vi "Host Gen Trajectory.vi"(7 "Trajectory Pattern":T3(ring)=enum."Centered", 8 "Depth Ctrl Array\n(% Thickness)":dbl[](array[numeric])=[20.0, 30.0, 40.0] min=10.0 max=90.0 step=5.0 format="%#_g%%", 9 "Traj Scale Radius from Pupil Radius (Between 0 and 1)":dbl, 10 "Traj Offset from Pupil Center [mm]":dbl[](array[numeric]), 11 "SCAN_NO":string="0000") -> (0 "zVisTraj":dbl[](array[numeric]) format="%_6g", 1 "yVisTraj":dbl[](array[numeric]) format="%_6g", 2 "xVisTraj":dbl[](array[numeric]) format="%_6g")   [LabVIEW 2016]
uses:
  <vilib>/silver_ctls/ArrayMatrixCluster/Real Matrix NI_Silver.ctl
  <vilib>/Analysis/Matrix/Datatypes/RealMatrix.ctl
  <vilib>/Analysis/7linalg.llb/Real Cholesky Factorization.vi
  <vilib>/Analysis/1siggen.llb/Ramp Pattern by Samples.vi
  <vilib>/Analysis/baseanly.llb/Mean (DBL).vi
  <vilib>/Analysis/baseanly.llb/Full Cholesky Factorization.vi
  <vilib>/Analysis/baseanly.llb/Full Real Matrix Cholesky Factorization.vi
  <vilib>/Analysis/BLAS.llb/dasum - Absolute Values Sum (DBL).vi
  <vilib>/Analysis/Matrix/Numeric/Conversions/Array To Matrix - RA2.vi
  <vilib>/Analysis/NI_AALBase.lvlib
  <vilib>/gmath/NI_Gmath.lvlib
  <vilib>/Analysis/NI_AALPro.lvlib
  <vilib>/Analysis/NI_AALBLAS.lvlib
  <vilib>/Analysis/Matrix/NI_Matrix.lvlib
panel:
  out "size(s)":i32
  out "L4_out":dbl[][](array[numeric])
  out "L3_out":dbl[][](array[numeric])
  out "L2_out":dbl[][](array[numeric])
  out "L1_out":dbl[][](array[numeric])
  out "Zi":dbl[][](array[numeric])
  out "Zp":dbl[][](array[numeric])
  out "Za":dbl[][](array[numeric])
  out "Y":dbl[][](array[numeric])
  out "X":dbl[][](array[numeric])
  out "x_out":dbl[][](array[numeric])
  out "y_out":dbl[][](array[numeric])
  out "z_out":dbl[][](array[numeric])
  out "Tool Rotation":dbl[][](array[numeric])
  out "vacf_out":dbl[][](array[numeric])
  out "time (at via pts)":dbl[][](array[numeric])
  in  "Tab Control":T1(tab)
  out "zi":dbl=5.0 format="%#_3g"
  out "zp_true":dbl=5.0 format="%#_3g"
  out "zp_work":dbl=5.0 format="%#_3g"
  out "za_work":dbl=5.0 format="%#_3g"
  out "za_true":dbl=5.0 format="%#_3g"
  in  "Reflective Index":dbl=1.35 format="%#_13g"
  out "Semi-Axes [mm]":T2
  out "Lens Thickness [mm]":dbl format="%#_3g"
  out "Iris Center [mm]":dbl[](array[numeric]) format="%#_3g"
  in  "Half Span Angle":dbl=60.0
  in  "Radial Attenuation":dbl=0.2 min=0.0 max=1.0 step=0.1
  in  "XY Safety Gap [mm]":dbl=1.5 format="%#_13g"
  out "Avg Iris z_coord [mm]":dbl=-2.0 format="%#_3g"
  in  "Cycle Time [sec]":dbl[](array[numeric])=[60.0, 90.0, 120.0]
  in  "Sampling Rate [Hz]":i32=1000
  out "Za Safety Gap [mm]":dbl[](array[numeric]) format="%#_3g"
  out "Zp Safety Gap [mm]":dbl[](array[numeric]) format="%#_3g"
  in  "No. of Lobes":dbl=10.0
  in  "Radial Offset":dbl=0.2 min=0.0 max=1.0
  in  "Dist Iris2Front [mm]":dbl[](array[numeric])=[0.1, 0.1, 0.1]
  out "No. of Cycles":i32
  out "Total Time [sec]":dbl
  out "Theta1 Waveform Graph":dbl[](graph)
  out "Theta2 Waveform Graph":dbl[](graph)
  out "Theta3 Waveform Graph":dbl[](graph)
  out "Theta4 Waveform Graph":dbl[](graph)
  in  "vac_bnd":dbl[](array[numeric])=[80.0, 100.0]
  in  "z_thld":dbl[](array[numeric])=[0.5, 2.0]
  out "Vacuum Waveform Graph":dbl[](graph)
  out "Ygrid":dbl[](array[numeric])
  out "Xgrid":dbl[](array[numeric])
  in  "OCT z_orgin [mm]":dbl format="%#_13g"
  in  "OCT z_cornea [mm]":dbl format="%#_13g"
  in  "OCT z_post [mm]":dbl format="%#_13g"
  out "Trajectory Length [mm]":dbl[](array[numeric])
  out "Traj Px Waveform Graph":dbl[](graph)
  out "Traj Py Waveform Graph":dbl[](graph)
  out "Traj Pz Waveform Graph":dbl[](graph)
  out "Theta4 Overlaid":dbl[][](graph)
  out "Theta3 Overlaid":dbl[][](graph)
  out "Theta2 Overlaid":dbl[][](graph)
  out "Theta1 Overlaid":dbl[][](graph)
  # "Modify Trajectory Center and Radius"
  # "Workspace Parameters"
  # "Top View:"
  # "Cross-Sectioned View:"
  # "No-fly Zone"
  # "Entry Site Pattern"
  # "Centered Pattern"
  # "Z Workspace"
  # "Temporal"
  # "OCT Settings"
  # "XY 2D Grid"
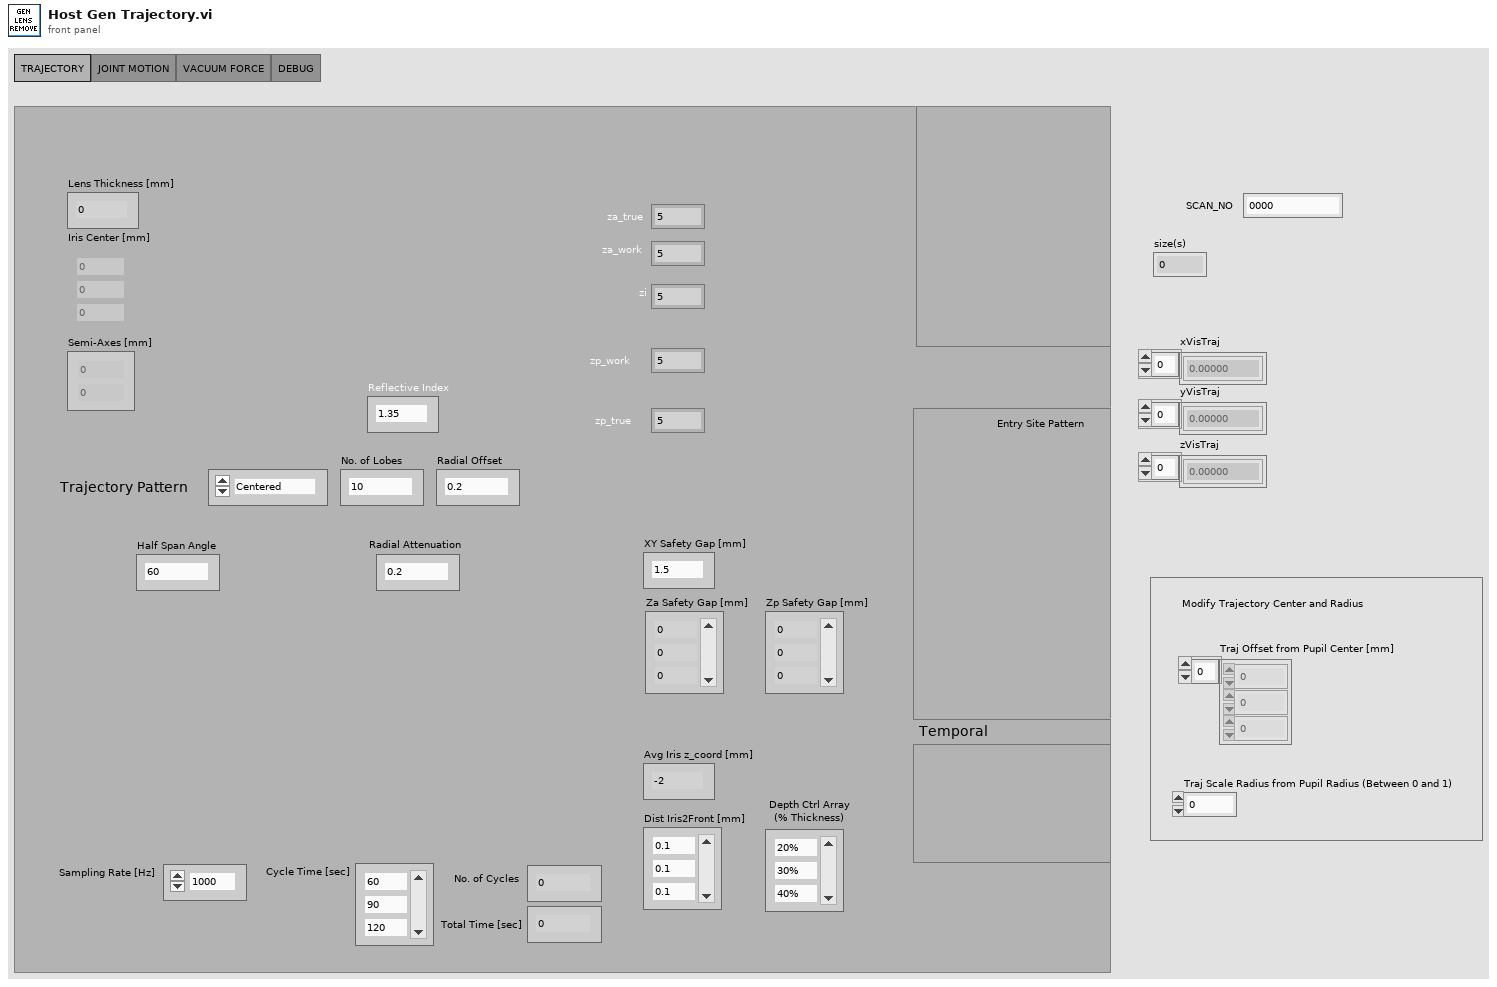
[diagram p1: front panel]
types:
  T1 = enum32{"TRAJECTORY", "JOINT MOTION", "VACUUM FORCE", "DEBUG"}
  T2 = typedef "Real Matrix NI_Silver.ctl" = dbl[][]
  T3 = enum16{"Entry Site", "Centered", "Insertion", "Extraction", "Reverse Entry Site", "Reverse Centered"}
  T4 = typedef "NI_Matrix.lvlib/RealMatrix.ctl" = dbl[][]
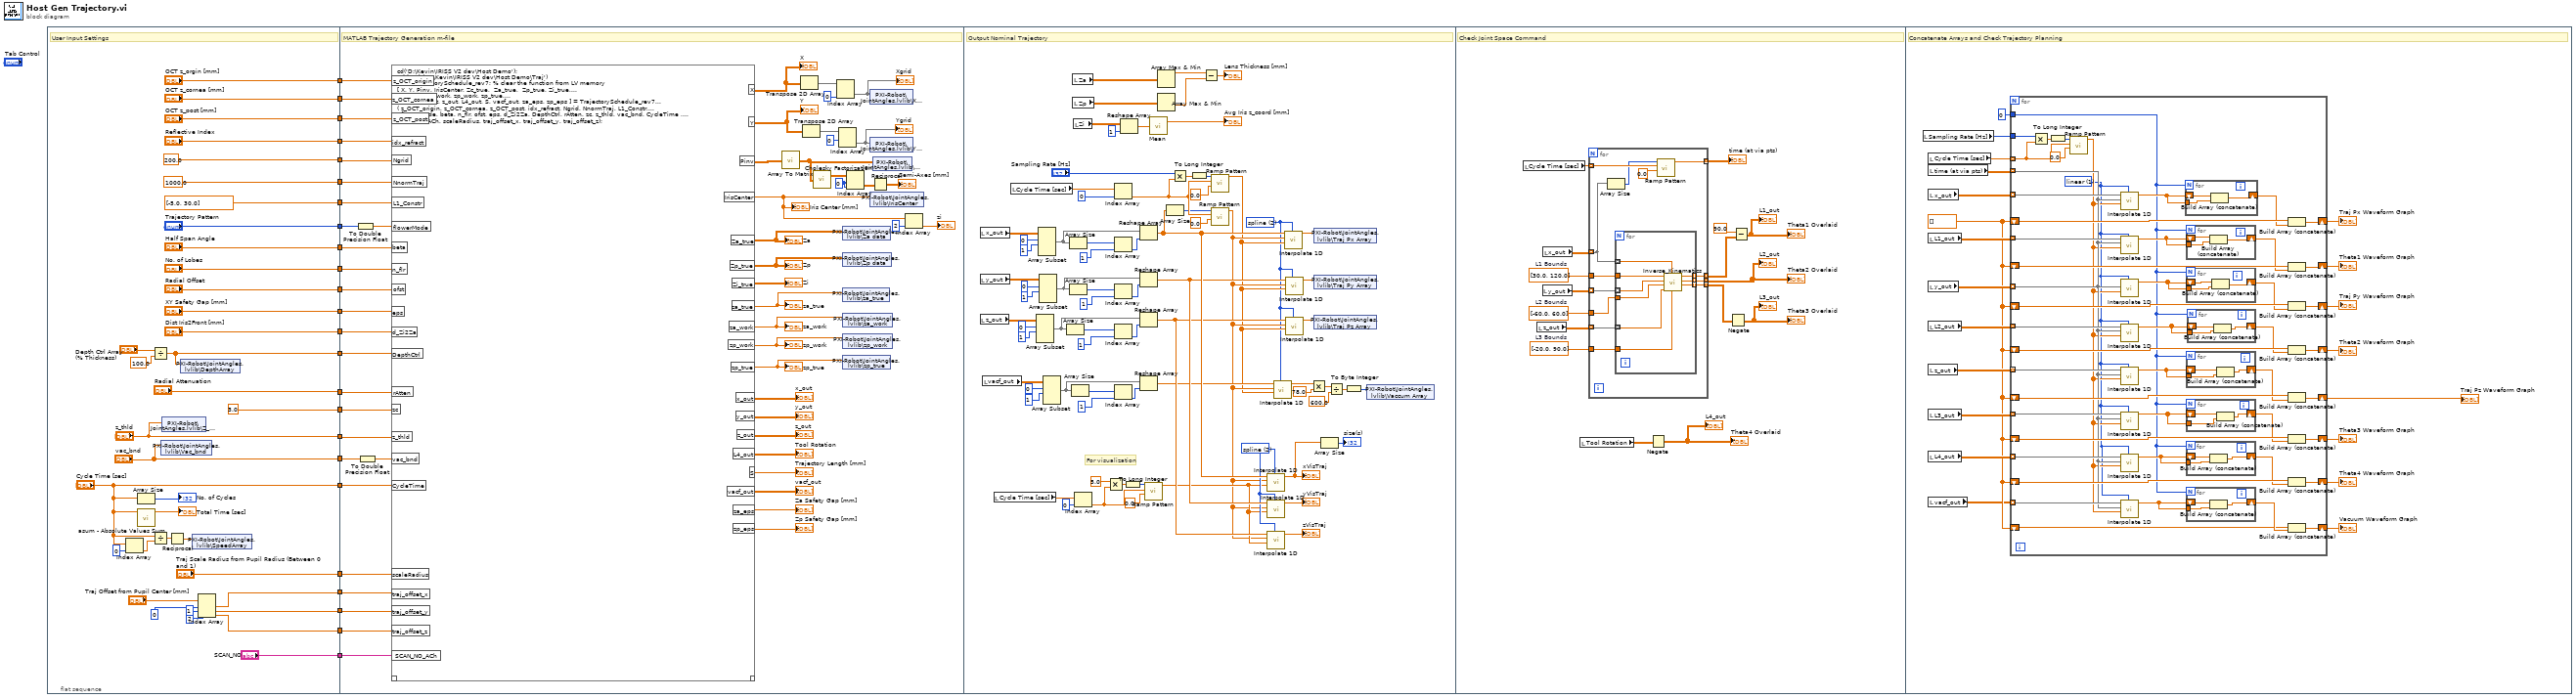
[diagram p0: block diagram]
diagram:
  n1 = flat-sequence {
    tunnel: [200.0 ("Real")] -> w24
    tunnel: ["No. of Lobes"] -> w23
    tunnel: ["Radial Offset"] -> w22
    tunnel: ["XY Safety Gap [mm]"] -> w21
    tunnel: ["Half Span Angle"] -> w20
    tunnel: [1000.0 ("Real")] -> w19
    tunnel: ["z_thld"] -> w18
    tunnel: ["vac_bnd"] -> w17
    tunnel: [3.0 ("zc")] -> w16
    tunnel: ["OCT z_orgin [mm]"] -> w15
    tunnel: ["OCT z_cornea [mm]"] -> w14
    tunnel: ["Reflective Index"] -> w13
    tunnel: ["Trajectory Pattern"] -> w12
    tunnel: ["Dist Iris2Front [mm]"] -> w11
    tunnel: [w36] -> w10
    tunnel: ["Radial Attenuation"] -> w9
    tunnel: ["OCT z_post [mm]"] -> w8
    tunnel: [dbl[] [-5.0, 30.0] ("z_thld")] -> w7
    tunnel: ["Cycle Time [sec]"] -> w6
    tunnel: ["SCAN_NO"] -> w5
    tunnel: ["Traj Scale Radius from Pupil Radius (Between 0 and 1)"] -> w4
    tunnel: [w30] -> w3
    tunnel: [w29] -> w2
    tunnel: [w28] -> w1
    tunnel: w24 -> [w114]
    tunnel: w23 -> [w118]
    tunnel: w22 -> [w117]
    tunnel: w21 -> [w116]
    tunnel: w20 -> [w108]
    tunnel: w19 -> [w104]
    tunnel: w18 -> [w103]
    tunnel: w17 -> [w101]
    tunnel: w16 -> [w99]
    tunnel: w15 -> [w97]
    tunnel: w14 -> [w96]
    tunnel: w13 -> [w95]
    tunnel: w12 -> [w94]
    tunnel: w11 -> [w86]
    tunnel: w10 -> [w87]
    tunnel: w9 -> [w92]
    tunnel: w8 -> [w88]
    tunnel: w7 -> [w83]
    tunnel: w6 -> [w81]
    tunnel: w5 -> [w65]
    tunnel: w4 -> [w64]
    tunnel: w3 -> [w63]
    tunnel: w2 -> [w62]
    tunnel: w1 -> [w61]
    frame #0 {
      # "User Input Settings"
      n2 = Index Array(array="Cycle Time [sec]", index=0) -> (element=w34:dbl)
      n3 = Array Size(array="Cycle Time [sec]") -> (size(s)=→"No. of Cycles":i32)
      n4 = call-poly <vilib>:"asum - Absolute Values Sum.vi"("x"="Cycle Time [sec]") -> ("dasum"=→"Total Time [sec]":dbl)  [unwired: 9 in, 1 out]
      n5 = Divide(x="Depth Ctrl Array\n(% Thickness)", y=100.0) -> (x/y=w36:dbl[])
      n6 = Divide(x="Cycle Time [sec]", y=w34) -> (x/y=w39:dbl[])
      n7 = shared-variable "PXI-Robot\\JointAngles.lvlib\\Vac_bnd"("vac_bnd") -> ()  [unwired: 1 in, 1 out]
      n8 = shared-variable "PXI-Robot\\JointAngles.lvlib\\Z_thld"("z_thld") -> ()  [unwired: 1 in, 1 out]
      n9 = Reciprocal(x=w39) -> (1/x=w38:dbl[])
      n10 = shared-variable "PXI-Robot\\JointAngles.lvlib\\DepthArray"(w36) -> ()  [unwired: 1 in, 1 out]
      n11 = shared-variable "PXI-Robot\\JointAngles.lvlib\\SpeedArray"(w38) -> ()  [unwired: 1 in, 1 out]
      n12 = Index Array(array="Traj Offset from Pupil Center [mm]", index #1=0 ("index"), index #2=1 ("index"), index #3=2 ("index")) -> (element #1=w30:dbl, element #2=w29:dbl, element #3=w28:dbl)
    }
    frame #1 {
      w77 = 0 ("index (row)")
      # "Outputs:\n% X: X 2D grid\n% Y: Y 2D grid\n% Pinv: inv(P) for XY ellipse representation\n% IrisCenter: 3-by-1 vector representing the center of iris\n% Zc_true: cornea surface\n% Za_true: anterior surface\n% Zp_true: posterior surface\n% Zi_true: iris plane\n% za_true: center z coordinate of AC\n% za_work: center z coordinate of workspace upper bound\n% zp_work: center z coordinate of workspace lower bound\n% zp_true: center z coordinate of PC\n% x_out: trajectory x position array\n% y_out: trajectory y position array\n% z_out: trajectory z position array\n% L4_out: tool rotation array\n% S: total arc length\n% vacf_out: vacuum scheduling array\n% za_eps: anterior safety gap\n% zp_eps: posterior safety gap\n\nInputs:\n% z_OCT_origin: where OCT performs 20-pt algorithm for coord. transformation\n% z_OCT_cornea: where OCT takes a snap shot for cornea\n% z_OCT_post: where OCT takes a snap shot for posterior capsule\n% idx_refract: refractive index\n% Ngrid: no. of XY grid points\n% Ntraj: no. of points used for trajectory generation\n% L1_Constr: constraint on L1 angles\n% flowerMode: flower pattern selection\n% beta: half angle range in deg on z=zi plane\n% n_flr: no. of lobes (even)\n% ofst: relative offset of flower pattern from starting point\n% eps:  safety gap thickness in XY in mm\n% d_Zi2Za: distance to anterior capsule\n% DepthCtrl: depth control in terms of thickness for each stage\n% zc: axis of aspiration points towards (0,~,zc)\n% z_thld: threshold z distances used to define extreme values of vacuum force\n% vac_bnd: extreme values of vacuum force\n% CycleTime: time elapsed per cycle"
      # "MATLAB Trajectory Generation m-file"
      n13 = To Double Precision Float(number=w94) -> (double precision float=w93:dbl)
      n14 = To Double Precision Float(number=w101) -> (double precision float=w100:dbl[])
      n15 = script code="cd('D:\\Kevin\\IRISS V2 dev\\Host Demo');\naddpath('D:\\Kevin\\IRISS V2 dev\\Host Demo\\Traj')\nclear TrajectorySchedule_rev7; % clear the function from LV memory\n[ X, Y, Pinv, IrisCenter, Zc_true,  Za_true,  Zp_true, Zi_true,...\n  za_true, za_work, zp_work, zp_true,...\n  x_out, y_out, z_out, L4_out, S, vacf_out, za_eps, zp_eps ] = TrajectorySchedule_rev7...\n( z_OCT_origin, z_OCT_cornea, z_OCT_post, idx_refract, Ngrid, NnormTraj, L1_Constr,...\n  flowerMode, beta, n_flr, ofst, eps, d_Zi2Za, DepthCtrl, rAtten, zc, z_thld, vac_bnd, CycleTime ,...\nSCAN_NO_ACh, scaleRadius, traj_offset_x, traj_offset_y, traj_offset_z);"("Ngrid"=w114, "n_flr"=w118, "ofst"=w117, "eps"=w116, "beta"=w108, "zc"=w99, "NnormTraj"=w104, "z_thld"=w103, "vac_bnd"=w100, "idx_refract"=w95, "z_OCT_cornea"=w96, "z_OCT_origin"=w97, "flowerMode"=w93, "d_Zi2Za"=w86, "DepthCtrl"=w87, "rAtten"=w92, "z_OCT_post"=w88, "L1_Constr"=w83, "CycleTime"=w81, "SCAN_NO_ACh"=w65, "scaleRadius"=w64, "traj_offset_x"=w63, "traj_offset_y"=w62, "traj_offset_z"=w61) -> ("x_out"=→"x_out":dbl[][], "y_out"=→"y_out":dbl[][], "z_out"=→"z_out":dbl[][], "S"=→"Trajectory Length [mm]":dbl[], "X"=w106:dbl[][], "Y"=w110:dbl[][], "Zp_true"=w98:dbl[][], "Za_true"=w105:dbl[][], "L4_out"=→"Tool Rotation":dbl[][], "vacf_out"=→"vacf_out":dbl[][], "Pinv"=w80:dbl[][], "IrisCenter"=w67:dbl[], "Zi_true"=→"Zi":dbl[][], "za_eps"=→"Za Safety Gap [mm]":dbl[], "zp_eps"=→"Zp Safety Gap [mm]":dbl[], "za_true"=w71:dbl, "za_work"=w70:dbl, "zp_work"=w69:dbl, "zp_true"=w68:dbl)  [unwired: 1 in, 1 out]
      "X" <- w106
      "Y" <- w110
      "Zp" <- w98
      "Za" <- w105
      "Iris Center [mm]" <- w67
      "za_true" <- w71
      "za_work" <- w70
      "zp_work" <- w69
      "zp_true" <- w68
      n16 = call-poly <vilib>:"Array To Matrix.vi"("Real 2D Array"=w80) -> ("Real Matrix"=w79:T4)
      n17 = Transpose 2D Array(2D array=w106) -> (transposed array=w113:dbl[][])
      n18 = Transpose 2D Array(2D array=w110) -> (transposed array=w111:dbl[][])
      n19 = call-poly <vilib>:"Cholesky Factorization.vi"("A"=w79) -> ("Cholesky"=w78:T4)  [unwired: 1 out]
      n20 = Index Array(array=w113, index (col)=0 ("disabled index (col)")) -> (element=w90:dbl[])  [unwired: 1 in]
      "Xgrid" <- w90
      n21 = Index Array(array=w111, index (row)=0 ("disabled index (col)")) -> (element=w89:dbl[])  [unwired: 1 in]
      "Ygrid" <- w89
      n22 = shared-variable "PXI-Robot\\JointAngles.lvlib\\Za data"(w105) -> ()  [unwired: 1 in, 1 out]
      n23 = shared-variable "PXI-Robot\\JointAngles.lvlib\\Zp data"(w98) -> ()  [unwired: 1 in, 1 out]
      n24 = shared-variable "PXI-Robot\\JointAngles.lvlib\\za_true"(w71) -> ()  [unwired: 1 in, 1 out]
      n25 = shared-variable "PXI-Robot\\JointAngles.lvlib\\za_work"(w70) -> ()  [unwired: 1 in, 1 out]
      n26 = shared-variable "PXI-Robot\\JointAngles.lvlib\\zp_work"(w69) -> ()  [unwired: 1 in, 1 out]
      n27 = shared-variable "PXI-Robot\\JointAngles.lvlib\\zp_true"(w68) -> ()  [unwired: 1 in, 1 out]
      n28 = Index Array(array=w78, index (row)=w77, index (col)=w77) -> (element=w76:T4)
      n29 = shared-variable "PXI-Robot\\JointAngles.lvlib\\IrisCenter"(w67) -> ()  [unwired: 1 in, 1 out]
      n30 = shared-variable "PXI-Robot\\JointAngles.lvlib\\X grid"(w90) -> ()  [unwired: 1 in, 1 out]
      n31 = shared-variable "PXI-Robot\\JointAngles.lvlib\\Y grid"(w89) -> ()  [unwired: 1 in, 1 out]
      n32 = Reciprocal(x=w76) -> (1/x=→"Semi-Axes [mm]":T4)
      n33 = shared-variable "PXI-Robot\\JointAngles.lvlib\\Pinv"(w79) -> ()  [unwired: 1 in, 1 out]
      n34 = Index Array(array=w67, index=2) -> (element=→"zi":dbl)
    }
    frame #2 {
      w147 = 2 items=["nearest", "linear", "spline", "cubic Hermite", "Lagrange"] ("method")
      w125 = 2 items=["nearest", "linear", "spline", "cubic Hermite", "Lagrange"] ("method")
      # "For visualization"
      # "Output Nominal Trajectory"
      n35 = local read "x_out"() -> (w179:dbl[][])
      n36 = local read "y_out"() -> (w178:dbl[][])
      n37 = local read "z_out"() -> (w156:dbl[][])
      n38 = local read "vacf_out"() -> (w135:dbl[][])
      n39 = local read "Cycle Time [sec]"() -> (w141:dbl[])
      n40 = local read "Cycle Time [sec]"() -> (w165:dbl[])
      n41 = Array Subset(array=w156, index (row)=0 ("index"), length (row)=1 ("length")) -> (w157:dbl[][])  [unwired: 2 in]
      n42 = Array Subset(array=w179, index (row)=0 ("index"), length (row)=1 ("length")) -> (w182:dbl[][])  [unwired: 2 in]
      n43 = Array Subset(array=w178, index (row)=0 ("index"), length (row)=1 ("length")) -> (w175:dbl[][])  [unwired: 2 in]
      n44 = Array Subset(array=w135, index (row)=0 ("index"), length (row)=1 ("length")) -> (w129:dbl[][])  [unwired: 2 in]
      n45 = Array Size(array=w157) -> (size(s)=w170:i32[])
      n46 = Array Size(array=w182) -> (size(s)=w181:i32[])
      n47 = Array Size(array=w175) -> (size(s)=w176:i32[])
      n48 = Array Size(array=w129) -> (size(s)=w132:i32[])
      n49 = local read "Za"() -> (w193:dbl[][])
      n50 = local read "Zp"() -> (w192:dbl[][])
      n51 = local read "Zi"() -> (w188:dbl[][])
      n52 = Index Array(array=w141, index=0) -> (element=w142:dbl)
      n53 = Multiply(x=5.0, y=w142) -> (x*y=w144:dbl)
      n54 = Index Array(array=w165, index=0) -> (element=w158:dbl)
      n55 = Index Array(array=w181, index=1) -> (element=w180:i32)
      n56 = Index Array(array=w176, index=1) -> (element=w177:i32)
      n57 = Index Array(array=w170, index=1) -> (element=w169:i32)
      n58 = Index Array(array=w132, index=1) -> (element=w130:i32)
      n59 = Reshape Array(w188, 1 ("dimension size")) -> (w186:dbl[])
      n60 = To Long Integer(number=w144) -> (32bit integer=w145:i32)
      n61 = Reshape Array(w182, w180) -> (w150:dbl[])
      n62 = Reshape Array(w175, w177) -> (w149:dbl[])
      n63 = Reshape Array(w157, w169) -> (w148:dbl[])
      n64 = Reshape Array(w129, w130) -> (w128:dbl[])
      n65 = call-poly <vilib>:"Ramp Pattern.vi"("start"=0.0, "end"=w142, "samples"=w145) -> ("Ramp Pattern"=w139:dbl[])  [unwired: 7 in, 1 out]
      n66 = call-poly <vilib>:"Mean.vi"("X"=w186) -> ("mean"=→"Avg Iris z_coord [mm]":dbl)  [unwired: 1 out]
      n67 = Array Max & Min(array=w193) -> (max value=w191:dbl)  [unwired: 3 out]
      n68 = Array Max & Min(array=w192) -> (min value=w190:dbl)  [unwired: 3 out]
      n69 = Array Size(array=w150) -> (size(s)=w155:i32)
      n70 = Multiply(x="Sampling Rate [Hz]", y=w158) -> (x*y=w161:dbl)
      n71 = To Long Integer(number=w161) -> (32bit integer=w162:i32)
      n72 = Subtract(x=w191, y=w190) -> (x-y=→"Lens Thickness [mm]":dbl)
      n73 = call-poly <vilib>:"Ramp Pattern.vi"("start"=0.0, "end"=w158, "samples"=w162) -> ("Ramp Pattern"=w126:dbl[])  [unwired: 7 in, 1 out]
      n74 = call-poly <vilib>:"Ramp Pattern.vi"("start"=0.0, "end"=w158, "samples"=w155) -> ("Ramp Pattern"=w127:dbl[])  [unwired: 7 in, 1 out]
      n75 = call <vilib>:"Interpolate 1D.vi"("method"=w147, "xi"=w139, "X"=w127, "Y"=w150) -> ("yi"=w136:dbl[])  [unwired: 5 in, 2 out]
      "xVisTraj" <- w136
      n76 = call <vilib>:"Interpolate 1D.vi"("method"=w147, "xi"=w139, "X"=w127, "Y"=w149) -> ("yi"=→"yVisTraj":dbl[])  [unwired: 5 in, 2 out]
      n77 = call <vilib>:"Interpolate 1D.vi"("method"=w147, "xi"=w139, "X"=w127, "Y"=w148) -> ("yi"=→"zVisTraj":dbl[])  [unwired: 5 in, 2 out]
      n78 = call <vilib>:"Interpolate 1D.vi"("method"=w125, "xi"=w126, "X"=w127, "Y"=w128) -> ("yi"=w119:dbl[])  [unwired: 5 in, 2 out]
      n79 = call <vilib>:"Interpolate 1D.vi"("method"=w125, "xi"=w126, "X"=w127, "Y"=w150) -> ("yi"=w153:dbl[])  [unwired: 5 in, 2 out]
      n80 = call <vilib>:"Interpolate 1D.vi"("method"=w125, "xi"=w126, "X"=w127, "Y"=w149) -> ("yi"=w154:dbl[])  [unwired: 5 in, 2 out]
      n81 = call <vilib>:"Interpolate 1D.vi"("method"=w125, "xi"=w126, "X"=w127, "Y"=w148) -> ("yi"=w152:dbl[])  [unwired: 5 in, 2 out]
      n82 = Multiply(x=w119, y=78.0 ("x")) -> (x*y=w122:dbl[])
      n83 = shared-variable "PXI-Robot\\JointAngles.lvlib\\Traj Px Array"(w153) -> ()  [unwired: 1 in, 1 out]
      n84 = shared-variable "PXI-Robot\\JointAngles.lvlib\\Traj Py Array"(w154) -> ()  [unwired: 1 in, 1 out]
      n85 = shared-variable "PXI-Robot\\JointAngles.lvlib\\Traj Pz Array"(w152) -> ()  [unwired: 1 in, 1 out]
      n86 = Array Size(array=w136) -> (size(s)=→"size(s)":i32)
      n87 = Divide(x=w122, y=600.0 ("x")) -> (x/y=w121:dbl[])
      n88 = To Byte Integer(number=w121) -> (8bit integer=w124:i8[])
      n89 = shared-variable "PXI-Robot\\JointAngles.lvlib\\Vaccum Array"(w124) -> ()  [unwired: 1 in, 1 out]
    }
    frame #3 {
      w207 = dbl[] [-20.0, 90.0]  # L3 Bounds
      w208 = dbl[] [-60.0, 60.0]  # L2 Bounds
      w209 = dbl[] [30.0, 120.0]  # L1 Bounds
      # "Check Joint Space Command"
      n90 = local read "Cycle Time [sec]"() -> (w194:dbl[])
      n91 = local read "z_out"() -> (w204:dbl[][])
      n92 = local read "y_out"() -> (w205:dbl[][])
      n93 = local read "x_out"() -> (w206:dbl[][])
      n94 = local read "Tool Rotation"() -> (w199:dbl[][])
      n95 = for {
        tunnel: w194 -> [w221] mode=indexing
        tunnel: w209 -> [w220]
        tunnel: w208 -> [w219]
        tunnel: w207 -> [w218]
        tunnel: w206 -> [w212] mode=indexing
        tunnel: w205 -> [w217] mode=indexing
        tunnel: w204 -> [w216] mode=indexing
        tunnel: [w215] -> w201 mode=indexing
        tunnel: [w214] -> w200 mode=indexing
        tunnel: [w213] -> w198 mode=indexing
        tunnel: [w210] -> w203 mode=indexing
        n96 = Array Size(array=w212) -> (size(s)=w211:i32)
        n97 = for {
          tunnel: w220 -> [w231]
          tunnel: w219 -> [w230]
          tunnel: w218 -> [w229]
          tunnel: w212 -> [w228] mode=indexing
          tunnel: w217 -> [w227] mode=indexing
          tunnel: w216 -> [w226] mode=indexing
          tunnel: [w225] -> w215 mode=indexing
          tunnel: [w224] -> w214 mode=indexing
          tunnel: [w223] -> w213 mode=indexing
          n98 = call "Inverse_Kinematics.vi"("B3"=w229, "px"=w228, "pz"=w226, "B2"=w230, "py"=w227, "B1"=w231) -> ("theta 3"=w223:dbl, "theta 2"=w224:dbl, "theta 1"=w225:dbl)  [unwired: 1 out]
        }
        n99 = call-poly <vilib>:"Ramp Pattern.vi"("start"=0.0, "end"=w221, "samples"=w211) -> ("Ramp Pattern"=w210:dbl[])  [unwired: 7 in, 1 out]
      }
      "L2_out" <- w200
      "time (at via pts)" <- w203
      "Theta2 Overlaid" <- w200
      n100 = Negate(x=w199) -> (-x=→"Theta4 Overlaid" →"L4_out":dbl[][])
      n101 = Negate(x=w198) -> (-x=→"L3_out" →"Theta3 Overlaid":dbl[][])
      n102 = Subtract(x=90.0, y=w201) -> (x-y=→"L1_out" →"Theta1 Overlaid":dbl[][])
    }
    frame #4 {
      w234 = dbl[] []
      # "Concatenate Arrays and Check Trajectory Planning"
      n103 = local read "Sampling Rate [Hz]"() -> (w235:i32)
      n104 = local read "Cycle Time [sec]"() -> (w250:dbl[])
      n105 = local read "time (at via pts)"() -> (w252:dbl[][])
      n106 = local read "x_out"() -> (w251:dbl[][])
      n107 = local read "L1_out"() -> (w249:dbl[][])
      n108 = local read "y_out"() -> (w248:dbl[][])
      n109 = local read "L2_out"() -> (w247:dbl[][])
      n110 = local read "z_out"() -> (w246:dbl[][])
      n111 = local read "L3_out"() -> (w245:dbl[][])
      n112 = local read "L4_out"() -> (w244:dbl[][])
      n113 = local read "vacf_out"() -> (w233:dbl[][])
      n114 = for {
        tunnel: w252 -> [w257] mode=indexing
        tunnel: w251 -> [w301] mode=indexing
        tunnel: w250 -> [w293] mode=indexing
        tunnel: w235 -> [w300]
        tunnel: w249 -> [w298] mode=indexing
        tunnel: w248 -> [w297] mode=indexing
        tunnel: w247 -> [w296] mode=indexing
        tunnel: w246 -> [w295] mode=indexing
        tunnel: w245 -> [w294] mode=indexing
        tunnel: w244 -> [w292] mode=indexing
        shift-right: [w281] -> w243
        shift-left: w234 -> [w282]
        shift-right: [w279] -> w242
        shift-left: w234 -> [w280]
        shift-right: [w277] -> w241
        shift-left: w234 -> [w278]
        shift-right: [w275] -> w240
        shift-left: w234 -> [w276]
        shift-right: [w273] -> w239
        shift-left: w234 -> [w274]
        shift-right: [w272] -> w238
        shift-left: w234 -> [w271]
        shift-right: [w270] -> w237
        shift-left: w234 -> [w269]
        tunnel: 0 ("No. of Cycles") -> [w253]
        shift-right: [w259] -> w232
        shift-left: w234 -> [w254]
        tunnel: w233 -> [w258] mode=indexing
        w255 = 1 items=["nearest", "linear", "spline", "cubic Hermite", "Lagrange"] ("method")
        n115 = Multiply(x=w300, y=w293) -> (x*y=w291:dbl)
        n116 = To Long Integer(number=w291) -> (32bit integer=w290:i32)
        n117 = call-poly <vilib>:"Ramp Pattern.vi"("start"=0.0, "end"=w293, "samples"=w290) -> ("Ramp Pattern"=w256:dbl[])  [unwired: 7 in, 1 out]
        n118 = call <vilib>:"Interpolate 1D.vi"("method"=w255, "xi"=w256, "X"=w257, "Y"=w301) -> ("yi"=w289:dbl[])  [unwired: 5 in, 2 out]
        n119 = call <vilib>:"Interpolate 1D.vi"("method"=w255, "xi"=w256, "X"=w257, "Y"=w298) -> ("yi"=w288:dbl[])  [unwired: 5 in, 2 out]
        n120 = call <vilib>:"Interpolate 1D.vi"("method"=w255, "xi"=w256, "X"=w257, "Y"=w297) -> ("yi"=w287:dbl[])  [unwired: 5 in, 2 out]
        n121 = call <vilib>:"Interpolate 1D.vi"("method"=w255, "xi"=w256, "X"=w257, "Y"=w296) -> ("yi"=w286:dbl[])  [unwired: 5 in, 2 out]
        n122 = call <vilib>:"Interpolate 1D.vi"("method"=w255, "xi"=w256, "X"=w257, "Y"=w295) -> ("yi"=w285:dbl[])  [unwired: 5 in, 2 out]
        n123 = call <vilib>:"Interpolate 1D.vi"("method"=w255, "xi"=w256, "X"=w257, "Y"=w294) -> ("yi"=w284:dbl[])  [unwired: 5 in, 2 out]
        n124 = call <vilib>:"Interpolate 1D.vi"("method"=w255, "xi"=w256, "X"=w257, "Y"=w292) -> ("yi"=w283:dbl[])  [unwired: 5 in, 2 out]
        n125 = call <vilib>:"Interpolate 1D.vi"("method"=w255, "xi"=w256, "X"=w257, "Y"=w258) -> ("yi"=w260:dbl[])  [unwired: 5 in, 2 out]
        n126 = for {
          N: w253 -> [_]
          shift-right: [w325] -> w262
          shift-left: w289 -> [w324]
          tunnel: w289 -> [w323]
          n127 = Build Array (concatenate)(w324, w323) -> (w325:dbl[])
        }
        n128 = for {
          N: w253 -> [_]
          tunnel: w283 -> [w306]
          shift-right: [w305] -> w263
          shift-left: w283 -> [w307]
          n129 = Build Array (concatenate)(w307, w306) -> (w305:dbl[])
        }
        n130 = for {
          N: w253 -> [_]
          tunnel: w260 -> [w303]
          shift-right: [w302] -> w261
          shift-left: w260 -> [w304]
          n131 = Build Array (concatenate)(w304, w303) -> (w302:dbl[])
        }
        n132 = for {
          N: w253 -> [_]
          shift-right: [w320] -> w268
          shift-left: w288 -> [w322]
          tunnel: w288 -> [w321]
          n133 = Build Array (concatenate)(w322, w321) -> (w320:dbl[])
        }
        n134 = for {
          N: w253 -> [_]
          shift-right: [w317] -> w267
          shift-left: w287 -> [w319]
          tunnel: w287 -> [w318]
          n135 = Build Array (concatenate)(w319, w318) -> (w317:dbl[])
        }
        n136 = for {
          N: w253 -> [_]
          shift-right: [w311] -> w265
          shift-left: w285 -> [w313]
          tunnel: w285 -> [w312]
          n137 = Build Array (concatenate)(w313, w312) -> (w311:dbl[])
        }
        n138 = for {
          N: w253 -> [_]
          shift-right: [w308] -> w264
          shift-left: w284 -> [w310]
          tunnel: w284 -> [w309]
          n139 = Build Array (concatenate)(w310, w309) -> (w308:dbl[])
        }
        n140 = for {
          N: w253 -> [_]
          shift-right: [w314] -> w266
          shift-left: w286 -> [w316]
          tunnel: w286 -> [w315]
          n141 = Build Array (concatenate)(w316, w315) -> (w314:dbl[])
        }
        n142 = Build Array (concatenate)(w282, w262) -> (w281:dbl[])
        n143 = Build Array (concatenate)(w280, w268) -> (w279:dbl[])
        n144 = Build Array (concatenate)(w278, w267) -> (w277:dbl[])
        n145 = Build Array (concatenate)(w276, w266) -> (w275:dbl[])
        n146 = Build Array (concatenate)(w274, w265) -> (w273:dbl[])
        n147 = Build Array (concatenate)(w271, w264) -> (w272:dbl[])
        n148 = Build Array (concatenate)(w269, w263) -> (w270:dbl[])
        n149 = Build Array (concatenate)(w254, w261) -> (w259:dbl[])
      }
      "Theta1 Waveform Graph" <- w242
      "Traj Px Waveform Graph" <- w243
      "Theta2 Waveform Graph" <- w240
      "Theta4 Waveform Graph" <- w237
      "Theta3 Waveform Graph" <- w238
      "Traj Py Waveform Graph" <- w241
      "Traj Pz Waveform Graph" <- w239
      "Vacuum Waveform Graph" <- w232
    }
  }
